vi "Windows to Linux Path.vi"(8 "error in (no error)":errorcluster, 11 "Windows path":string) -> (0 "error out":errorcluster, 3 "Linux Path":string)   [LabVIEW 2019, in "BlueTOMLSerializer.lvlib"]
uses:
  BlueTOMLSerializer.lvlib
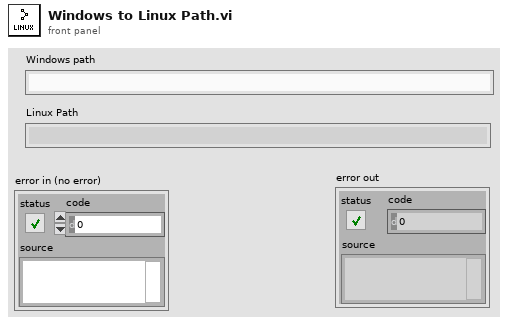
[diagram p1: front panel]
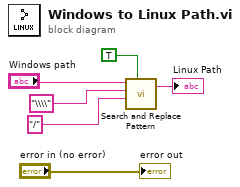
[diagram p0: block diagram]
diagram:
  n1 = call <vilib>:"Search and Replace Pattern.vi"("string"="Windows path", "regular expression (\"\")"="\\\\" ("regular expression (\"\")"), "replace string (\"\")"="/" ("replace string (\"\")"), "replace all? (F)"=TRUE) -> ("result string"=→"Linux Path":string)  [unwired: 1 in, 1 out]
  "error out" <- "error in (no error)"
